vi "vector_v0.vi"() -> ()   [LabVIEW 2009]
panel:
  out "Vector LED-uri":bool[](array[boolean])=[TRUE, FALSE, TRUE, FALSE, TRUE, FALSE, TRUE, TRUE]
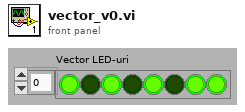
[diagram p1: front panel]
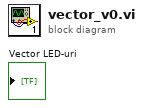
[diagram p0: block diagram]
diagram:
